vi "FRC Color and Shape Processing Example.vi"() -> ()   [LabVIEW 2025]
uses:
  <vilib>/Rock Robotics/WPI/Camera/WPI_CameraSettings Read MJPG.ctl
  <vilib>/Rock Robotics/WPI/Camera/WPI_CameraImageSize.ctl
  Vision Support Code/Camera Types.ctl
  <vilib>/vision/Pattern Matching.llb/IMAQ Match Range Setting.ctl
  <vilib>/vision/Pattern Matching.llb/IMAQ Curve Parameters.ctl
  <vilib>/vision/NI_Vision_Development_Module.lvlib
panel:
  out "Template":T1(plugin-control)
  in  "Camera Type":T2=enum."MS HD3000 square"
  in  "Image Path":path=path "Sample Images/KicoffFilmingVision"
  in  "image files":string[](array[string])
  out "Detected Totes":T3(array[cluster]) {"Normalized Rect"."Numeric 5" format="%#_2g"; "Normalized Rect"."Numeric 3" format="%#_2g"; "Normalized Rect"."Numeric 2" format="%#_2g"; "Normalized Rect"."Numeric" format="%#_2g"}
  in  "Score Threshold":dbl=75.0
  in  "Source":enum32{"Files", "Camera"}(tab)
  in  "Images":i32(listbox)
  in  "Folder Location":path=path "Sample Images"
  in  "Camera Settings":T4={"fps"=20, "compression"=30, "Image Size"=enum."320x240", "Config Shown"=FALSE}
  in  "Camera Address":string="USB 1"
  in  "Annotate":bool=TRUE
  out "ms to process":u32
  out "Sorted Scores":T6(array[cluster]) {"Correlation" format="%#_3g"; "Scale %" format="%#_3g"; "Score" format="%#_3g"}
  out "Particles":i32
  in  "Tote Color":T7={"Hue"={23.67058792990901, 48.923317529462665}, "Sat"={66.78571428571429, 255.0}, "Val"={48.571428571428584, 255.0}} {"Hue" scale=0.0..255.0 scale format="%#_3g"}
  out "Masked":T1(plugin-control)
  out "Original Image":T1(plugin-control)
  # "Instructions:\nUse Source to select image files from a directory or use a USB or IP camera connected to your laptop.\nUse Tote Color for initial processing, then search for the trained template image. Use Vision Assistant\nto train for different images or to modify Range Settings. \nThis example is effective within a few feet. It is likely not the right choice for distant patterns.\nAnnotations show the rectangle and the scores from top to bottom."
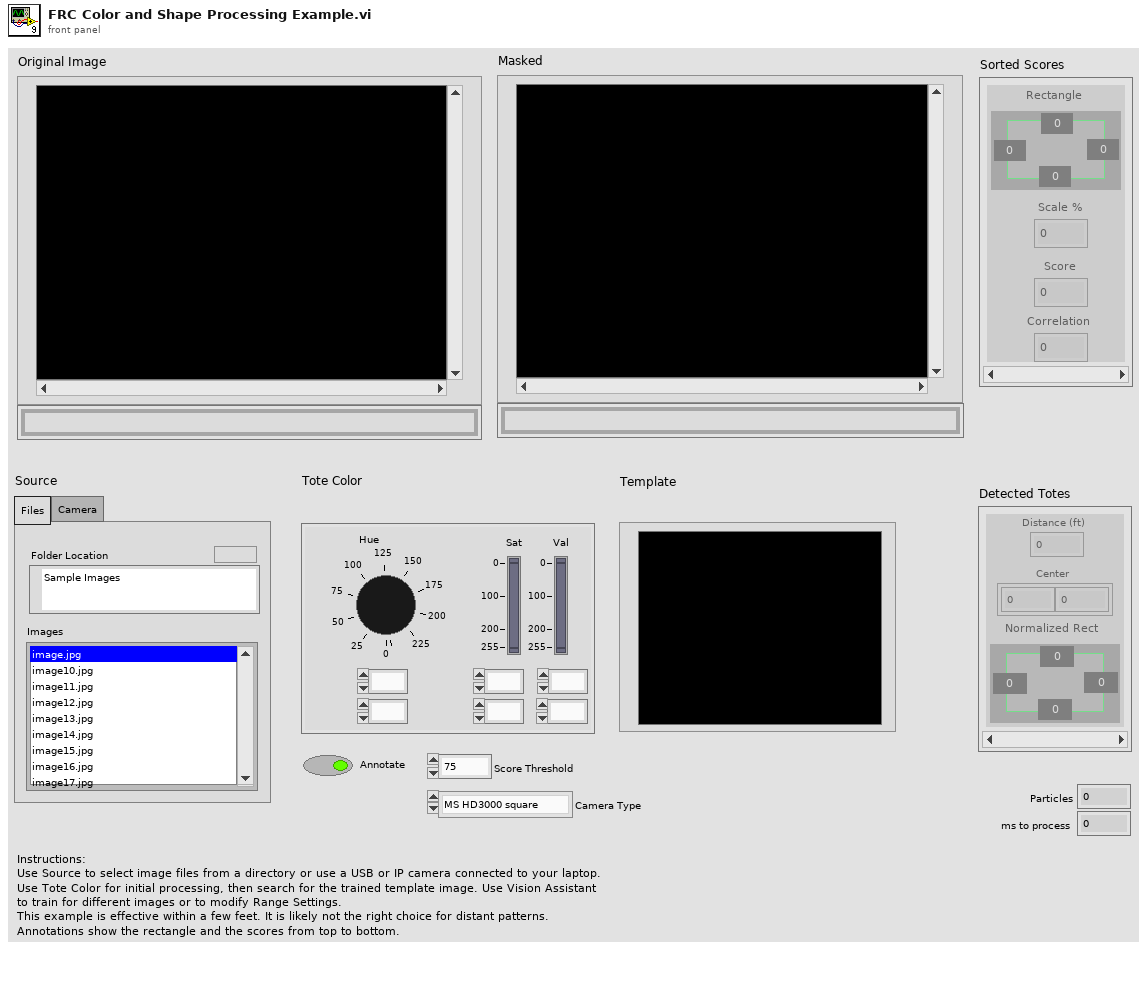
[diagram p1: front panel]
types:
  T1 = typedef "IMAQ Image.ctl" = refnum<image>
  T2 = typedef "Camera Types.ctl" = enum16{"206", "1011", "1013", "MS HD3000 square", "MS HD3000 640x480"}
  T3 = cluster{"Distance (ft)":dbl, "Center":cluster{dbl, dbl}, "Normalized Rect":cluster{"Numeric":dbl, "Numeric 2":dbl, "Numeric 3":dbl, "Numeric 5":dbl}}[]
  T4 = typedef "WPI_CameraSettings Read MJPG.ctl" = cluster{"fps":i32, "compression":i32, "Image Size":T5, "Config Shown":bool}
  T5 = typedef "WPI_CameraImageSize.ctl" = enum16{"640x480", "320x240", "160x120", "Custom"}
  T6 = cluster{"Rectangle":cluster{"Numeric":dbl, "Numeric 2":dbl, "Numeric 3":dbl, "Numeric 5":dbl}, "Scale %":dbl, "Score":dbl, "Correlation":dbl}[]
  T7 = cluster{"Hue":cluster{dbl, dbl}, "Sat":cluster{dbl, dbl}, "Val":cluster{dbl, dbl}}
  T8 = cluster{"Rotation":bool, "Scale":bool, "Occlusion":bool, "Reserved":bool, "Reserved":bool, "Reserved":bool}
  T9 = typedef "IMAQ Curve Parameters.ctl" = cluster{"Extraction Mode":u32, "Edge Threshold":i32, "Edge Filter Size":u32, "Min Length":i32, "Row Search Step Size":i32, "Col Search Step Size":i32, "Max Endpoint Gap":i32, "Closed":bool, "Subpixel":bool}
  T10 = typedef "IMAQ Match Range Setting.ctl" = cluster{"Match Constraints":u32, "Min":dbl, "Max":dbl}
  T11 = typedef "Image Type" = u32
  T12 = typedef "Particle Parameters" = i32
  T13 = cluster{"[0]":dbl, "[1]":dbl, "[2]":dbl, "[3]":dbl}
  T14 = cluster{"[0]":dbl, "[1]":dbl, "[2]":dbl, "[3]":dbl, "[4]":dbl}
  T15 = typedef "ROI Descriptor" = cluster{"Global Rectangle":i32[], "Contours":cluster{"ID":enum32{"External", "Internal"}, "Type":u32, "Coordinates":i32[]}[]}
  T16 = typedef "IMAQ GM Match Report.ctl" = cluster{"Position":cluster{"x":sgl, "y":sgl}, "Angle":sgl, "Scale":sgl, "Score":sgl, "Bounding Box":cluster{"x":sgl, "y":sgl}[], "Contrast Reversed":bool, "Occlusion %":sgl, "Template Target Curve Score":sgl, "Target Template Curve Score":sgl, "Correlation Score":sgl}
  T17 = cluster{cluster{"[0]":dbl, "[1]":dbl, "[2]":dbl, "[3]":dbl}, "Position":cluster{"x":sgl, "y":sgl}, "Bounding Box":cluster{"x":sgl, "y":sgl}[], "Scale":sgl, "Score":sgl, "Correlation Score":sgl}
  T18 = cluster{"Rectangle":cluster{"Numeric":dbl, "Numeric 2":dbl, "Numeric 3":dbl, "Numeric 5":dbl}, "Scale":dbl, "Score":dbl, "Correlation":dbl}[]
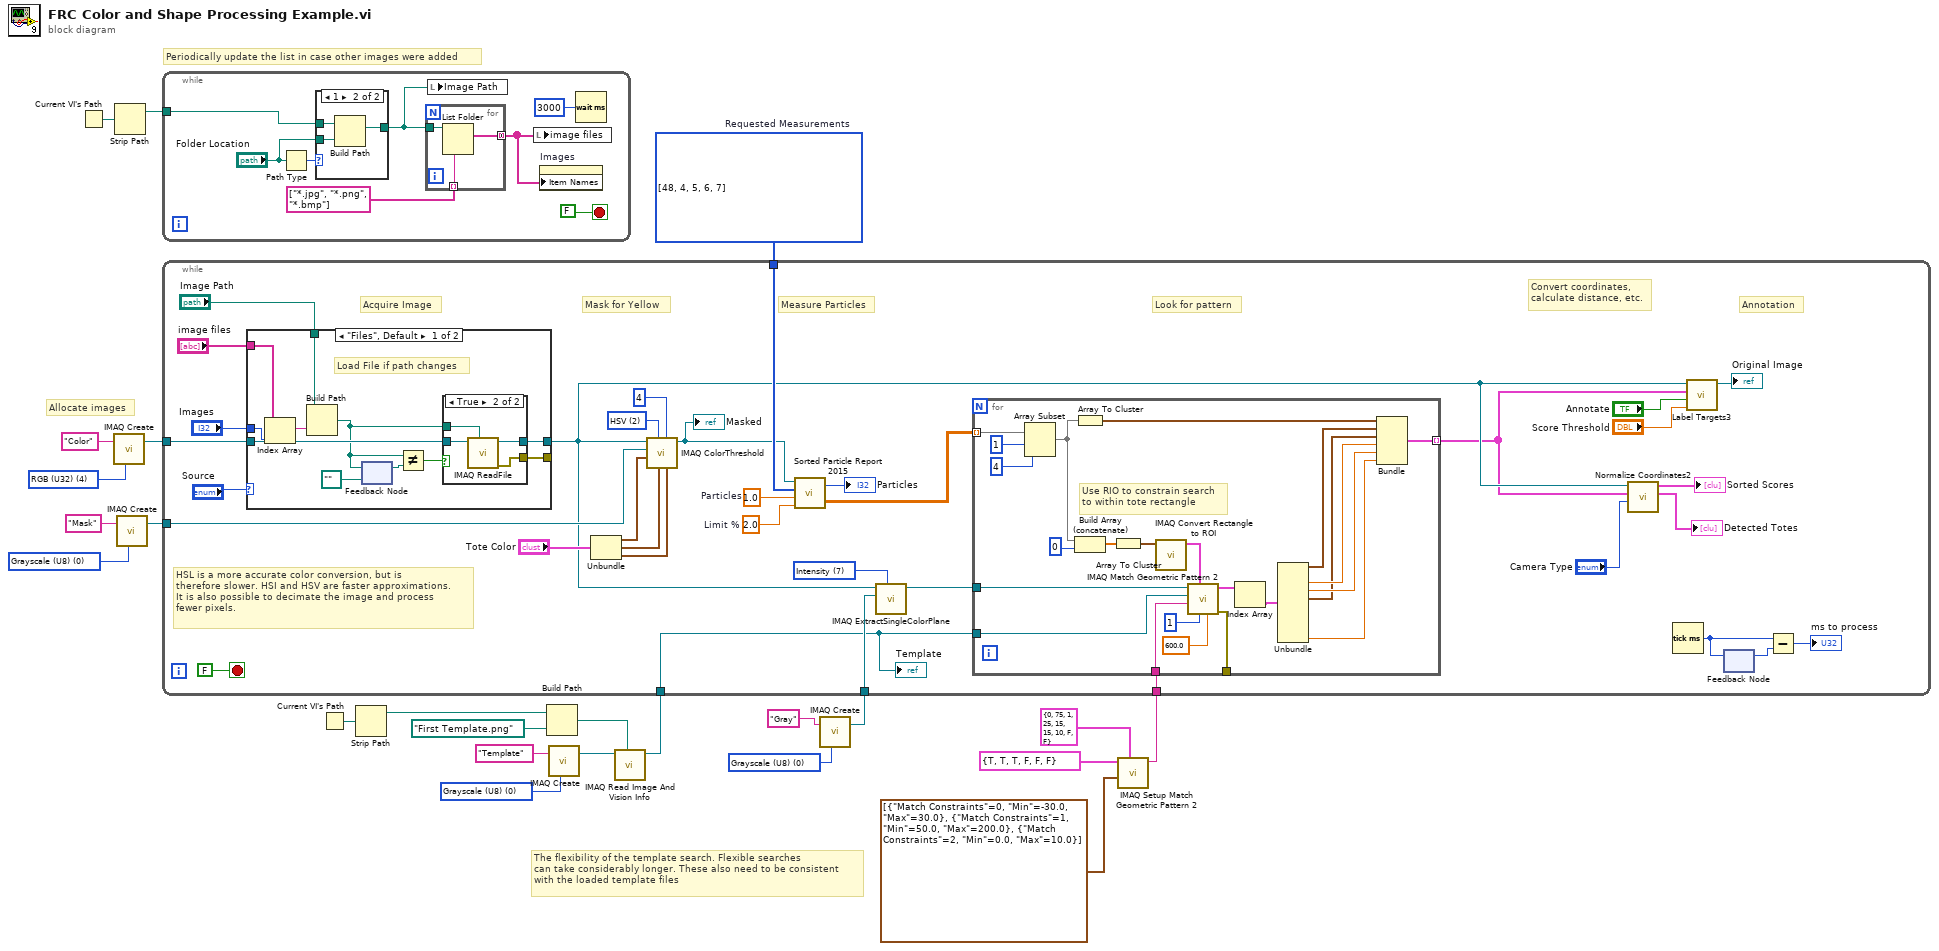
[diagram p0: block diagram]
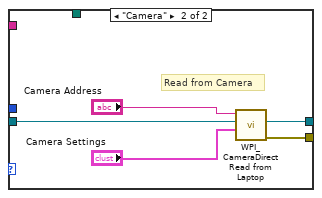
[diagram p4: hidden frame]
diagram:
  w13 = T11 0 items=["Grayscale (U8)", "Grayscale (I16)", "Grayscale (SGL)", "Complex (CSG)", "RGB (U32)", "HSL (U32)", "RGB (U64)", "Grayscale (U16)"] ("Image Type")
  w15 = T11 0 items=["Grayscale (U8)", "Grayscale (I16)", "Grayscale (SGL)", "Complex (CSG)", "RGB (U32)", "HSL (U32)", "RGB (U64)", "Grayscale (U16)"] ("Image Type")
  w18 = T12[] [48, 4, 5, 6, 7] items=["Center of Mass X", "Center of Mass Y", "First Pixel X", "First Pixel Y", "Bounding Rect Left", "Bounding Rect Top", "Bounding Rect Right", "Bounding Rect Bottom", "Max Feret Diameter Start X", "Max Feret Diameter Start Y", "Max Feret Diameter End X", "Max Feret Diameter End Y", "Max Horiz. Segment Length Left", "Max Horiz. Segment Length Right", "Max Horiz. Segment Length Row", "-", "Bounding Rect Width", "Bounding Rect Height", "Bounding Rect Diagonal", "Perimeter", "Convex Hull Perimeter", "Holes' Perimeter", "Max Feret Diameter", "Equivalent Ellipse Major Axis", "Equivalent Ellipse Minor Axis", "Equivalent Ellipse Minor Axis (Feret)", "Equivalent Rect Long Side", "Equivalent Rect Short Side", "Equivalent Rect Diagonal", "Equivalent Rect Short Side (Feret)", "Average Horiz. Segment Length", "Average Vert. Segment Length", "Hydraulic Radius", "Waddel Disk Diameter", "-", "Area", "Holes' Area", "Particle & Holes' Area", "Convex Hull Area", "Image Area", "-", "Number of Holes", "Number of Horiz. Segments", "Number of Vert. Segments", "-", "Orientation", "Max Feret Diameter Orientation", "-", "% Area/Image Area", "% Area/(Particle & Holes' Area)", "Ratio of Equivalent Ellipse Axes", "Ratio of Equivalent Rect Sides", "-", "Elongation Factor", "Compactness Factor", "Heywood Circularity Factor", "Type Factor", "-", "Sum X", "Sum Y", "Sum XX", "Sum XY", "Sum YY", "Sum XXX", "Sum XXY", "Sum XYY", "Sum YYY", "-", "Moment of Inertia XX", "Moment of Inertia XY", "Moment of Inertia YY", "Moment of Inertia XXX", "Moment of Inertia XXY", "Moment of Inertia XYY", "Moment of Inertia YYY", "Norm. Moment of Inertia XX", "Norm. Moment of Inertia XY", "Norm. Moment of Inertia YY", "Norm. Moment of Inertia XXX", "Norm. Moment of Inertia XXY", "Norm. Moment of Inertia XYY", "Norm. Moment of Inertia YYY", "Hu Moment 1", "Hu Moment 2", "Hu Moment 3", "Hu Moment 4", "Hu Moment 5", "Hu Moment 6", "Hu Moment 7"]  # Requested Measurements
  w21 = T11 0 items=["Grayscale (U8)", "Grayscale (I16)", "Grayscale (SGL)", "Complex (CSG)", "RGB (U32)", "HSL (U32)", "RGB (U64)", "Grayscale (U16)"] ("Image Type")
  w23 = T11 4 items=["Grayscale (U8)", "Grayscale (I16)", "Grayscale (SGL)", "Complex (CSG)", "RGB (U32)", "HSL (U32)", "RGB (U64)", "Grayscale (U16)"] ("Image Type")
  # "The flexibility of the template search. Flexible searches\ncan take considerably longer. These also need to be consistent\nwith the loaded template files"
  # "Periodically update the list in case other images were added"
  # "Allocate images"
  n1 = Current VI's Path() -> (path=w17:path)
  n2 = call "IMAQ Create"("Image Name"="Color", "Image Type"=w23) -> ("New Image"=w22:T1)  [unwired: 2 in, 2 out]
  n3 = Strip Path(path=w17) -> (stripped path=w16:path)  [unwired: 1 out]
  n4 = call "IMAQ Create"("Image Name"="Mask", "Image Type"=w21) -> ("New Image"=w19:T1)  [unwired: 2 in, 2 out]
  n5 = while {
    tunnel: w16 -> [w26]
    stop <- FALSE stop-if-true
    n6 = Path Type(1:"Folder Location") -> (0:w28:i16)
    n7 = case shown="1" w28 {
      tunnel: "Folder Location" -> [w33 w36]
      tunnel: [w33 w34] -> w25
      tunnel: w26 -> [_ w35]
      frame 0, Default {
      }
      frame 1 {
        n8 = Build Path(base path=w35, name or relative path=w36) -> (appended path=w34:path)
      }
    }
    n9 = for {
      tunnel: [w39] -> w29 mode=concatenating
      tunnel: w25 -> [w38]
      tunnel: string[] ["*.jpg", "*.png", "*.bmp"] -> [w37] mode=indexing
      n10 = List Folder(path=w38, pattern=w37) -> (filenames=w39:string[])  [unwired: 2 in, 3 out]
    }
    n11 = local write "Image Path"(w25) -> ()
    n12 = local write "image files"(w29) -> ()
    n13 = property on="Images" class="LstBox (strict)"("Item Names"=w29) -> ()  [unwired: 2 in, 2 out]
    n14 = Wait (ms)(milliseconds to wait=u32 3000) -> ()  [unwired: 1 out]
  }
  n15 = Current VI's Path() -> (path=w2:path)
  n16 = Strip Path(path=w2) -> (stripped path=w1:path)  [unwired: 1 out]
  n17 = Build Path(base path=w1, name or relative path=path "First Template.png") -> (appended path=w3:path)
  n18 = call "IMAQ Create"("Image Name"="Template", "Image Type"=w13) -> ("New Image"=w5:T1)  [unwired: 2 in, 2 out]
  n19 = call "IMAQ Read Image And Vision Info"("File Path"=w3, "Image"=w5) -> ("Image Out"=w4:T1)  [unwired: 2 in, 7 out]
  n20 = call "IMAQ Create"("Image Name"="Gray", "Image Type"=w15) -> ("New Image"=w7:T1)  [unwired: 2 in, 2 out]
  n21 = call "IMAQ Setup Match Geometric Pattern 2"("Curve Parameters"=T9 {"Extraction Mode"=0, "Edge Threshold"=75, "Edge Filter Size"=1, "Min Length"=25, "Row Search Step Size"=15, "Col Search Step Size"=15, "Max Endpoint Gap"=10, "Closed"=FALSE, "Subpixel"=FALSE}, "Range Settings"=T10[] [{"Match Constraints"=0, "Min"=-30.0, "Max"=30.0}, {"Match Constraints"=1, "Min"=50.0, "Max"=200.0}, {"Match Constraints"=2, "Min"=0.0, "Max"=10.0}], "Match Mode"=T8 {"Rotation"=TRUE, "Scale"=TRUE, "Occlusion"=TRUE, "Reserved"=FALSE, "Reserved"=FALSE, "Reserved"=FALSE}) -> ("Match Geometric Pattern 2 Setup Data"=w8:string)  [unwired: 7 in, 1 out]
  n22 = while {
    tunnel: w22 -> [w73]
    tunnel: w19 -> [w71]
    tunnel: w18 -> [w65]
    tunnel: w8 -> [w52]
    tunnel: w7 -> [w50]
    tunnel: w4 -> [w40]
    stop <- FALSE stop-if-true
    w54 = 7 items=["Red", "Green", "Blue", "Hue", "Saturation", "Luminance", "Value", "Intensity"] ("Color Plane")
    w62 = 2.0  # Limit %
    w64 = 1.0  # Particles
    w70 = u16 2 items=["RGB", "HSL", "HSV", "HSI"] ("Color Mode")
    # "Convert coordinates,\ncalculate distance, etc."
    # "Annotation"
    # "Measure Particles"
    # "Look for pattern"
    # "Mask for Yellow"
    # "Acquire Image"
    # "HSL is a more accurate color conversion, but is\ntherefore slower. HSI and HSV are faster approximations.\nIt is also possible to decimate the image and process\nfewer pixels."
    n23 = case shown="\"Files\", Default" "Source" {
      tunnel: [w107 w118] -> _
      tunnel: [w108 w117] -> w45
      tunnel: w73 -> [w106 w116]
      tunnel: "image files" -> [w98 _]
      tunnel: "Images" -> [w105 _]
      tunnel: "Image Path" -> [w103 _]
      frame "Files", Default {
        # "Load File if path changes"
        n24 = Index Array(array=w98, index=w105) -> (element=w104:string)
        n25 = Build Path(base path=w103, name or relative path=w104) -> (appended path=w99:path)
        n26 = feedback-in #1(w99) -> ()
        n27 = feedback #1(path "" ("appended path")) -> (w101:path)
        n28 = Not Equal?(x=w99, y=w101) -> (x != y?=w102:bool)
        n29 = case shown="True" w102 {
          tunnel: [w109 w113] -> w108
          tunnel: [_ w112] -> w107
          tunnel: w106 -> [w109 w111]
          tunnel: w99 -> [_ w110]
          frame False {
          }
          frame True {
            n30 = call "IMAQ ReadFile"("File Path"=w110, "Image"=w111) -> ("error out"=w112:errorcluster, "Image Out"=w113:T1)  [unwired: 5 in, 3 out]
          }
        }
      }
      frame "Camera" {
        # "Read from Camera"
        n31 = call <vilib>:"WPI_CameraDirect Read from Laptop.vi"("Camera Settings"="Camera Settings", "Image"=w116, "address"="Camera Address") -> ("error out"=w118:errorcluster, "Image Out"=w117:T1)  [unwired: 7 in]
      }
    }
    n32 = Unbundle("Tote Color") -> ("Hue"=w69:cluster{dbl, dbl}, "Sat"=w68:cluster{dbl, dbl}, "Val"=w67:cluster{dbl, dbl})
    n33 = call "IMAQ ColorThreshold"("Blue or Luma or Val or Inten Range"=w67, "Replace Value"=4, "Green or Sat Range"=w68, "Color Mode"=w70, "Red or Hue Range"=w69, "Image Dst"=w71, "Image Src"=w45) -> ("Image Dst Out"=w53:T1)  [unwired: 3 in, 1 out]
    "Masked" <- w53
    n34 = call "Sorted Particle Report 2015.vi"("Min Area Size %"=w62, "Particle Count Limit"=w64, "Pixel Measurements"=w65, "Image in"=w53) -> ("Sorted Data"=w49:dbl[][], "Particles"=→"Particles":i32)
    n35 = call "IMAQ ExtractSingleColorPlane"("Color Plane"=w54, "Image Dst"=w50, "Image Src"=w45) -> ("Image Dst Out"=w51:T1)  [unwired: 7 in, 1 out]
    n36 = for {
      tunnel: w49 -> [w95] mode=indexing
      tunnel: [w94] -> w44 mode=indexing
      tunnel: w51 -> [w85]
      tunnel: w52 -> [w87]
      tunnel: w40 -> [w77]
      tunnel: [w76] -> _
      # "Use RIO to constrain search\nto within tote rectangle"
      n37 = Array Subset(array=w95, index=1, length=4) -> (w88:dbl[])
      n38 = Array To Cluster(array=w88) -> (cluster=w89:T13)
      n39 = Build Array (concatenate)(w88, 0 ("length")) -> (w92:dbl[])
      n40 = Array To Cluster(array=w92) -> (cluster=w91:T14)
      n41 = call "IMAQ Convert Rectangle to ROI"("Rectangle"=w91) -> ("ROI Descriptor"=w90:T15)  [unwired: 8 in, 1 out]
      n42 = call "IMAQ Match Geometric Pattern 2"("Minimum Match Score"=sgl 600.0, "Number of Matches Requested"=1 ("Minimum Match Score"), "ROI Descriptor"=w90, "Match Geometric Pattern 2 Setup Data"=w87, "Template Image"=w77, "Image"=w85) -> ("error out"=w76:errorcluster, "Matches (pixel)"=w83:T16[])  [unwired: 2 in, 2 out]
      n43 = Index Array(array=w83) -> (element=w82:T16)  [unwired: 1 in]
      n44 = Unbundle(w82) -> ("Position"=w81:cluster{"x":sgl, "y":sgl}, "Scale"=w80:sgl, "Score"=w79:sgl, "Bounding Box"=w75:cluster{"x":sgl, "y":sgl}[], "Correlation Score"=w78:sgl)  [unwired: 5 out]
      n45 = Bundle(w89, "Position"=w81, "Bounding Box"=w75, "Scale"=w80, "Score"=w79, "Correlation Score"=w78) -> (w94:T17)  [unwired: 1 in]
    }
    n46 = call "Normalize Coordinates2.vi"("Camera Type"="Camera Type", "Targets"=w44, "Image in"=w45) -> ("Found Totes"=→"Detected Totes":T3, "Sorted Scores"=→"Sorted Scores":T18)  [unwired: 7 in]
    n47 = Tick Count (ms)() -> (millisecond timer value=w60:u32)
    n48 = call "Label Targets3.vi"("Score Threshold"="Score Threshold", "Annotate"="Annotate", "Targets"=w44, "Image in"=w45) -> ("Image out"=→"Original Image":T1)  [unwired: 7 in]
    n49 = feedback-in #2(w60) -> ()
    n50 = feedback #2() -> (w61:u32)  [unwired: 1 in]
    n51 = Subtract(x=w60, y=w61) -> (x-y=→"ms to process":u32)
    "Template" <- w40
  }
